vi "Coord window-Enable column name edit option.vi"(6 "Clicked on empty row":bool, 8 "error in (no error)":errorcluster, 9 "Cell Position":T1, 11 "Menu in":refnum<k9>) -> (0 "error out":errorcluster, 3 "Menu out":refnum<k9>)   [LabVIEW 2013]
uses:
  <vilib>/Utility/miscctls.llb/LVRowAndColumnTypeDef.ctl
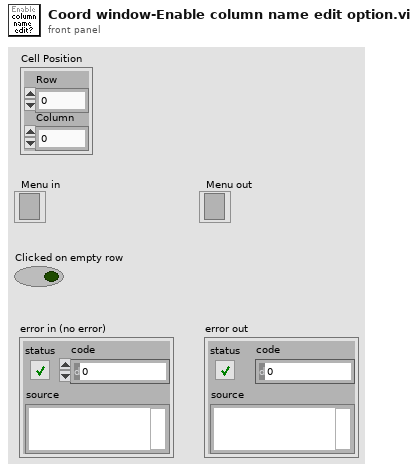
[diagram p1: front panel]
types:
  T1 = typedef "LVRowAndColumnTypeDef.ctl" = cluster{"Row":i32, "Column":i32}
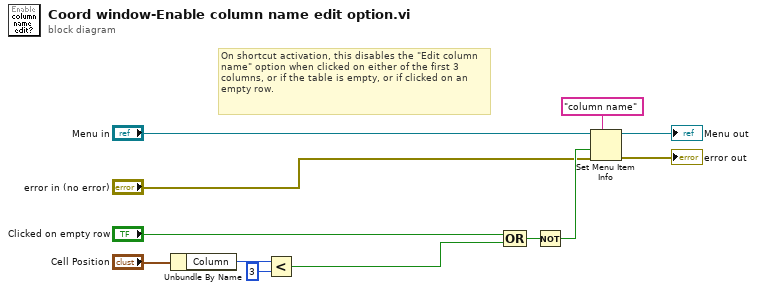
[diagram p0: block diagram]
diagram:
  # "On shortcut activation, this disables the \"Edit column name\" option when clicked on either of the first 3 columns, or if the table is empty, or if clicked on an empty row."
  n1 = Unbundle By Name("Cell Position") -> ("Column"=w8:i32)
  n2 = Less?(x=w8, y=3) -> (x < y?=w6:bool)
  n3 = Compound Arithmetic op=OR("Clicked on empty row", w6) -> (w5:bool)
  n4 = Not(x=w5) -> (.not. x?=w4:bool)
  n5 = Set Menu Item Info(7:"column name" ("item tag"), 8:"error in (no error)", 9:w4, 11:"Menu in") -> (0:→"error out":errorcluster, 3:→"Menu out":refnum<k9>)  [unwired: 3 in]
